vi "Receiver.vi"() -> ()   [LabVIEW 2021]
panel:
  out "String":string
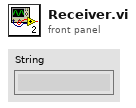
[diagram p1: front panel]
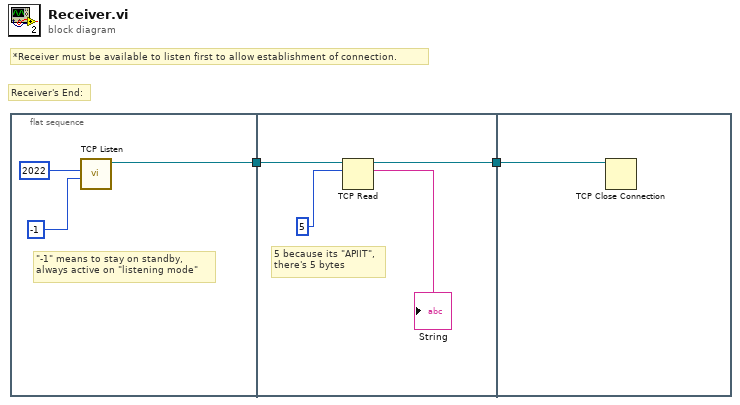
[diagram p0: block diagram]
diagram:
  # "*Receiver must be available to listen first to allow establishment of connection."
  # "Receiver's End:"
  n1 = flat-sequence {
    tunnel: [w3] -> w2
    tunnel: w2 -> [w9]
    tunnel: [w6] -> w1
    tunnel: w1 -> [w10]
    frame #0 {
      # "\"-1\" means to stay on standby, \nalways active on \"listening mode\""
      n2 = call <vilib>:"TCP Listen.vi"("timeout ms (wait forever: -1)"=-1, "port"=2022) -> ("connection ID"=w3:refnum<k5>)  [unwired: 5 in, 4 out]
    }
    frame #1 {
      # "5 because its \"APIIT\",\nthere's 5 bytes"
      n3 = TCP Read(connection ID=w9, bytes to read=5) -> (connection ID out=w6:refnum<k5>, data out=→"String":string)  [unwired: 3 in, 1 out]
    }
    frame #2 {
      n4 = TCP Close Connection(connection ID=w10) -> ()  [unwired: 2 in, 2 out]
    }
  }
